vi "hello.vi"() -> ()   [LabVIEW 2021]
panel:
  out "Boolean 2":bool
  in  "Boolean":bool
  out "String":string
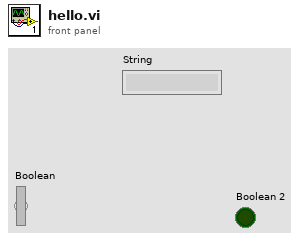
[diagram p1: front panel]
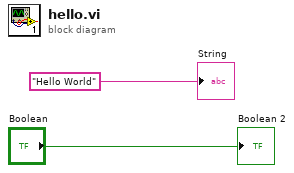
[diagram p0: block diagram]
diagram:
  "String" <- "Hello World"
  "Boolean 2" <- "Boolean"
